vi "svx_Timebase Legend Visible.vi"(7 "Bounds In":T1, 8 "Prev Legend Visible":bool, 9 "Legend Visible":bool, 10 "Legend Width":u32) -> (5 "Bounds Out":T1)   [LabVIEW 2017, in "SVX Timebase.xctl"]
uses:
  <vilib>/addons/_XControls/Timebase Plot/SVX Timebase.xctl
  <vilib>/addons/_XControls/Timebase Plot/subVIs/svx_Timebase Bounds.ctl
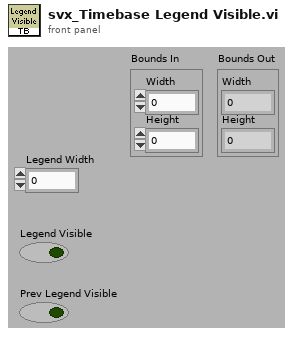
[diagram p1: front panel]
types:
  T1 = typedef "SVX Timebase.xctl/svx_Timebase Bounds.ctl" = cluster{"Width":u32, "Height":u32}
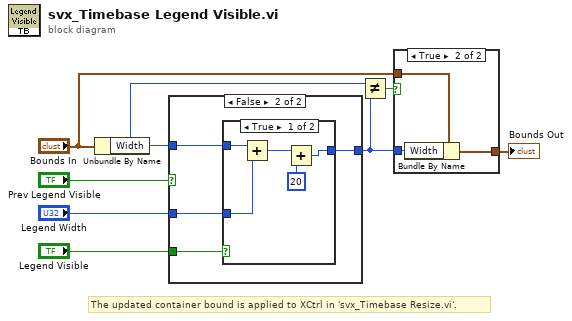
[diagram p0: block diagram]
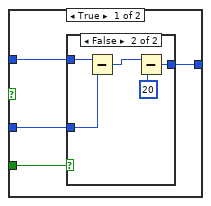
[diagram p3: hidden frame]
diagram:
  # "The updated container bound is applied to XCtrl in 'svx_Timebase Resize.vi'."
  n1 = Unbundle By Name("Bounds In") -> ("Width"=w3:u32)
  n2 = case shown="False" "Prev Legend Visible" {
    tunnel: "Legend Visible" -> [w9 w19]
    tunnel: "Legend Width" -> [w12 w22]
    tunnel: [w11 w21] -> w4
    tunnel: w3 -> [w10 w20]
    frame True {
      n3 = case shown="False" w9 {
        tunnel: w10 -> [w13 w18]
        tunnel: w12 -> [_ w17]
        tunnel: [w13 w16] -> w11
        frame True {
        }
        frame False {
          n4 = Subtract(x=w18, y=w17) -> (x-y=w15:u32)
          n5 = Subtract(x=w15, y=u32 20) -> (x-y=w16:u32)
        }
      }
    }
    frame False {
      n6 = case shown="True" w19 {
        tunnel: w20 -> [w27 w28]
        tunnel: w22 -> [w26 _]
        tunnel: [w24 w28] -> w21
        frame True {
          n7 = Add(x=w27, y=w26) -> (x+y=w25:u32)
          n8 = Add(x=w25, y=u32 20) -> (x+y=w24:u32)
        }
        frame False {
        }
      }
    }
  }
  n9 = Not Equal?(x=w3, y=w4) -> (x != y?=w5:bool)
  n10 = case shown="True" w5 {
    tunnel: w4 -> [_ w32]
    tunnel: "Bounds In" -> [w29 w31]
    tunnel: [w29 w30] -> w1
    frame False {
    }
    frame True {
      n11 = Bundle By Name(cluster=w31, "Width"=w32) -> (w30:T1)
    }
  }
  "Bounds Out" <- w1
